vi "TimerFGV.vi"(7 "Action":T1(ring), 8 "error in (no error)":errorcluster, 11 "Target Time (s)":dbl) -> (0 "error out":errorcluster, 1 "Time Elapsed (s)":dbl, 2 "Is Paused?":bool, 3 "Is Time Elapsed?":bool)   [LabVIEW 2024]
doc: "Generic Timer Functional Global Variable.\n\n\n--------\nPaulo Rossi\nprossi@aurumautomation.ca\n©2024 Aurum Automation Inc.\nOpen-Sourced per GNU GPL v3\n\nYou should have received a copy of the GNU General Public License along with this program. If not, see <https://www.gnu.org/licenses/>."
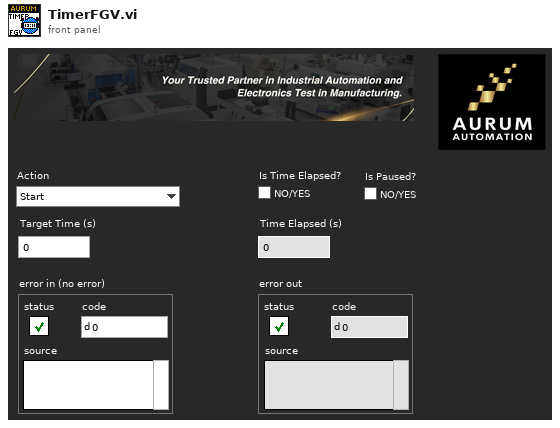
[diagram p1: front panel]
types:
  T1 = enum16{"Start", "Stop", "Reset", "Get Time Elapsed"}
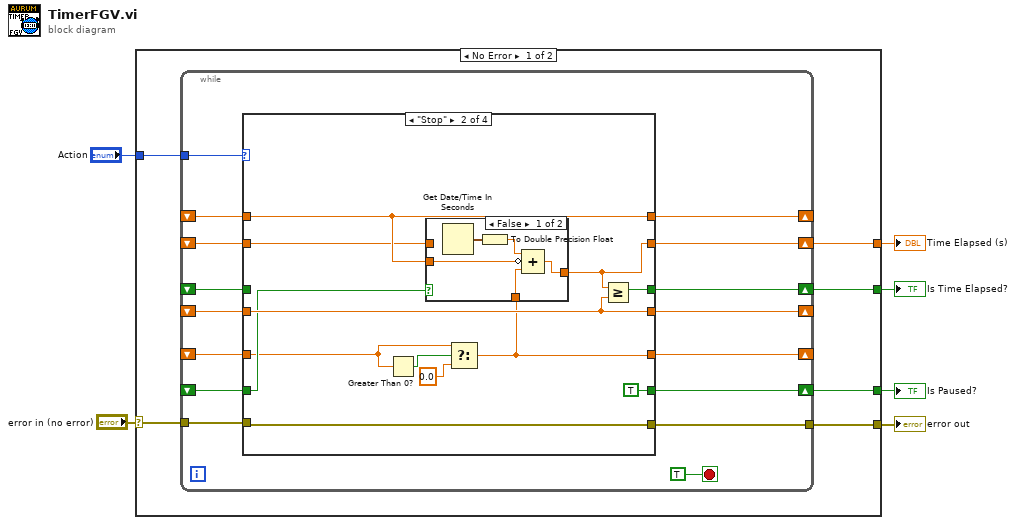
[diagram p0: block diagram]
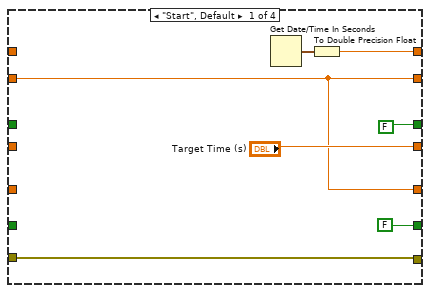
[diagram p2: hidden frame]
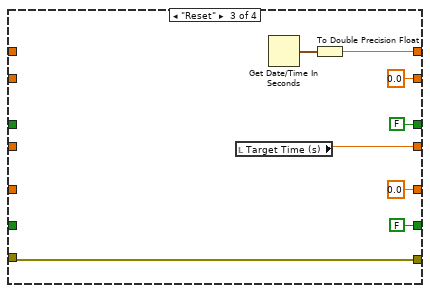
[diagram p4: hidden frame]
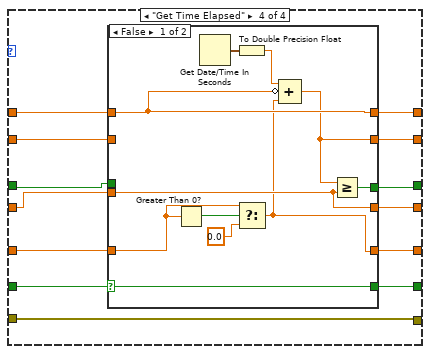
[diagram p5: hidden frame]
diagram:
  n1 = case shown="No Error" "error in (no error)" {
    selector: "error in (no error)" -> [w11 w92]
    tunnel: [w10 w92] -> w5
    tunnel: "Action" -> [w12 _]
    tunnel: [w9 _] -> w3
    tunnel: [w8 _] -> w2
    tunnel: [w7 _] -> w1
    frame No Error {
      n2 = while {
        tunnel: w12 -> [w27]
        shift-right: [w26] -> _
        shift-left: _ -> [w19]
        tunnel: w11 -> [w22]
        tunnel: [w21] -> w10
        shift-right: [w23] -> w9
        shift-left: _ -> [w15]
        shift-right: [w25] -> w8
        shift-left: _ -> [w16]
        shift-right: [w24] -> w7
        shift-left: _ -> [w20]
        shift-right: [w17] -> _
        shift-left: _ -> [w18]
        shift-right: [w14] -> _
        shift-left: _ -> [w13]
        stop <- TRUE stop-if-true
        n3 = case shown="\"Stop\"" w27 {
          tunnel: [w30 w45 w57 w68] -> w26
          tunnel: [FALSE ("Is Time Elapsed?") w43 FALSE ("Is Time Elapsed?") w72] -> w25
          tunnel: [w29 w40 0.0 ("Time Elapsed") w73] -> w24
          tunnel: [FALSE ("Is Time Elapsed?") TRUE ("Is Time Elapsed?") FALSE ("Is Time Elapsed?") w64] -> w23
          tunnel: [w33 w46 w56 w71] -> w21
          tunnel: w22 -> [w33 w46 w56 w71]
          tunnel: w20 -> [w29 w41 _ w67]
          tunnel: w19 -> [_ w45 _ w74]
          tunnel: w18 -> [_ w44 _ w70]
          tunnel: ["Target Time (s)" w44 w55 w66] -> w17
          tunnel: w16 -> [_ _ _ w65]
          tunnel: w15 -> [_ w42 _ w69]
          tunnel: [w29 w37 0.0 w62] -> w14
          tunnel: w13 -> [_ w36 _ w63]
          frame "Start", Default {
            n4 = Get Date/Time In Seconds() -> (seconds since 1Jan1904=w31:timestamp)
            n5 = To Double Precision Float(number=w31) -> (double precision float=w30:dbl)
          }
          frame "Stop" {
            n6 = Greater Than 0?(x=w36) -> (x > 0?=w38:bool)
            n7 = Select(t=w36, s=w38, f=0.0) -> (s? t:f=w37:dbl)
            n8 = case shown="False" w42 {
              tunnel: w45 -> [w50 _]
              tunnel: [w49 w53] -> w40
              tunnel: w41 -> [_ w53]
              tunnel: w37 -> [w48 _]
              frame False {
                n9 = Get Date/Time In Seconds() -> (seconds since 1Jan1904=w51:timestamp)
                n10 = To Double Precision Float(number=w51) -> (double precision float=w52:dbl)
                n11 = Compound Arithmetic op=ADD(w52, invert w50, w48) -> (w49:dbl)
              }
              frame True {
              }
            }
            n12 = Greater Or Equal?(x=w40, y=w44) -> (x >= y?=w43:bool)
          }
          frame "Reset" {
            n13 = local read "Target Time (s)"() -> (w55:dbl)
            n14 = Get Date/Time In Seconds() -> (seconds since 1Jan1904=w58:timestamp)
            n15 = To Double Precision Float(number=w58) -> (double precision float=w57:dbl)
          }
          frame "Get Time Elapsed" {
            n16 = case shown="False" w69 {
              selector: w69 -> [w80 w87]
              tunnel: w74 -> [w82 w91]
              tunnel: [w79 w90] -> w73
              tunnel: [w83 w88] -> w72
              tunnel: w70 -> [w81 w89]
              tunnel: [w82 w91] -> w68
              tunnel: w67 -> [_ w90]
              tunnel: [w81 w89] -> w66
              tunnel: w65 -> [_ w88]
              tunnel: [w80 w87] -> w64
              tunnel: w63 -> [w77 w86]
              tunnel: [w75 w86] -> w62
              frame False {
                n17 = Greater Than 0?(x=w77) -> (x > 0?=w76:bool)
                n18 = Get Date/Time In Seconds() -> (seconds since 1Jan1904=w84:timestamp)
                n19 = To Double Precision Float(number=w84) -> (double precision float=w85:dbl)
                n20 = Select(t=w77, s=w76, f=0.0) -> (s? t:f=w75:dbl)
                n21 = Compound Arithmetic op=ADD(w85, invert w82, w75) -> (w79:dbl)
                n22 = Greater Or Equal?(x=w79, y=w81) -> (x >= y?=w83:bool)
              }
              frame True {
              }
            }
          }
        }
      }
    }
    frame Error {
    }
  }
  "error out" <- w5
  "Is Paused?" <- w3
  "Is Time Elapsed?" <- w2
  "Time Elapsed (s)" <- w1
